vi "display.vi"() -> ()   [LabVIEW 2014]
uses:
  global variable.vi
  DataSocket/Read PLC Vars/Read U32 Var.vi
panel:
  out "选项卡控件":enum32{"选项卡 1", "选项卡 2", "选项卡 3"}(tab)
  out "Reject":i32
  out "FTT(%)":dbl format="%.1f%%"
  out "Pass":i32
  out "Actual":i32
  out "Target":dbl
  out "BTS(%)":dbl format="%.1f%%"
  out "Plan":dbl
  out "日期字符串":string
  out "时间字符串":string
  out "产品":string
  in  "生产状态":string="生产状态/Production Status"
  out "柱状图":cluster{"X轴":dbl[], "每小时产量":dbl[]}[](graph)
  out "日期字符串 2":string
  out "时间字符串 2":string
  out "产线":string
  out "日期字符串 3":string
  out "时间字符串 3":string
  out "C101":string="L541"
  out "V254":string="C53F"
  out "C101车型":string="S90L"
  out "FS11":string="CS11"
  out "FS11车型":string="领克03"
  out "V254车型":string="智道U7"
  out "FA1":string="FA1"
  # "/"
  # "/"
  # "/"
  # "/"
  # "/"
  # "/"
  # "/"
  # "/"
  # "/"
  # "/"
  # "/"
  # "/"
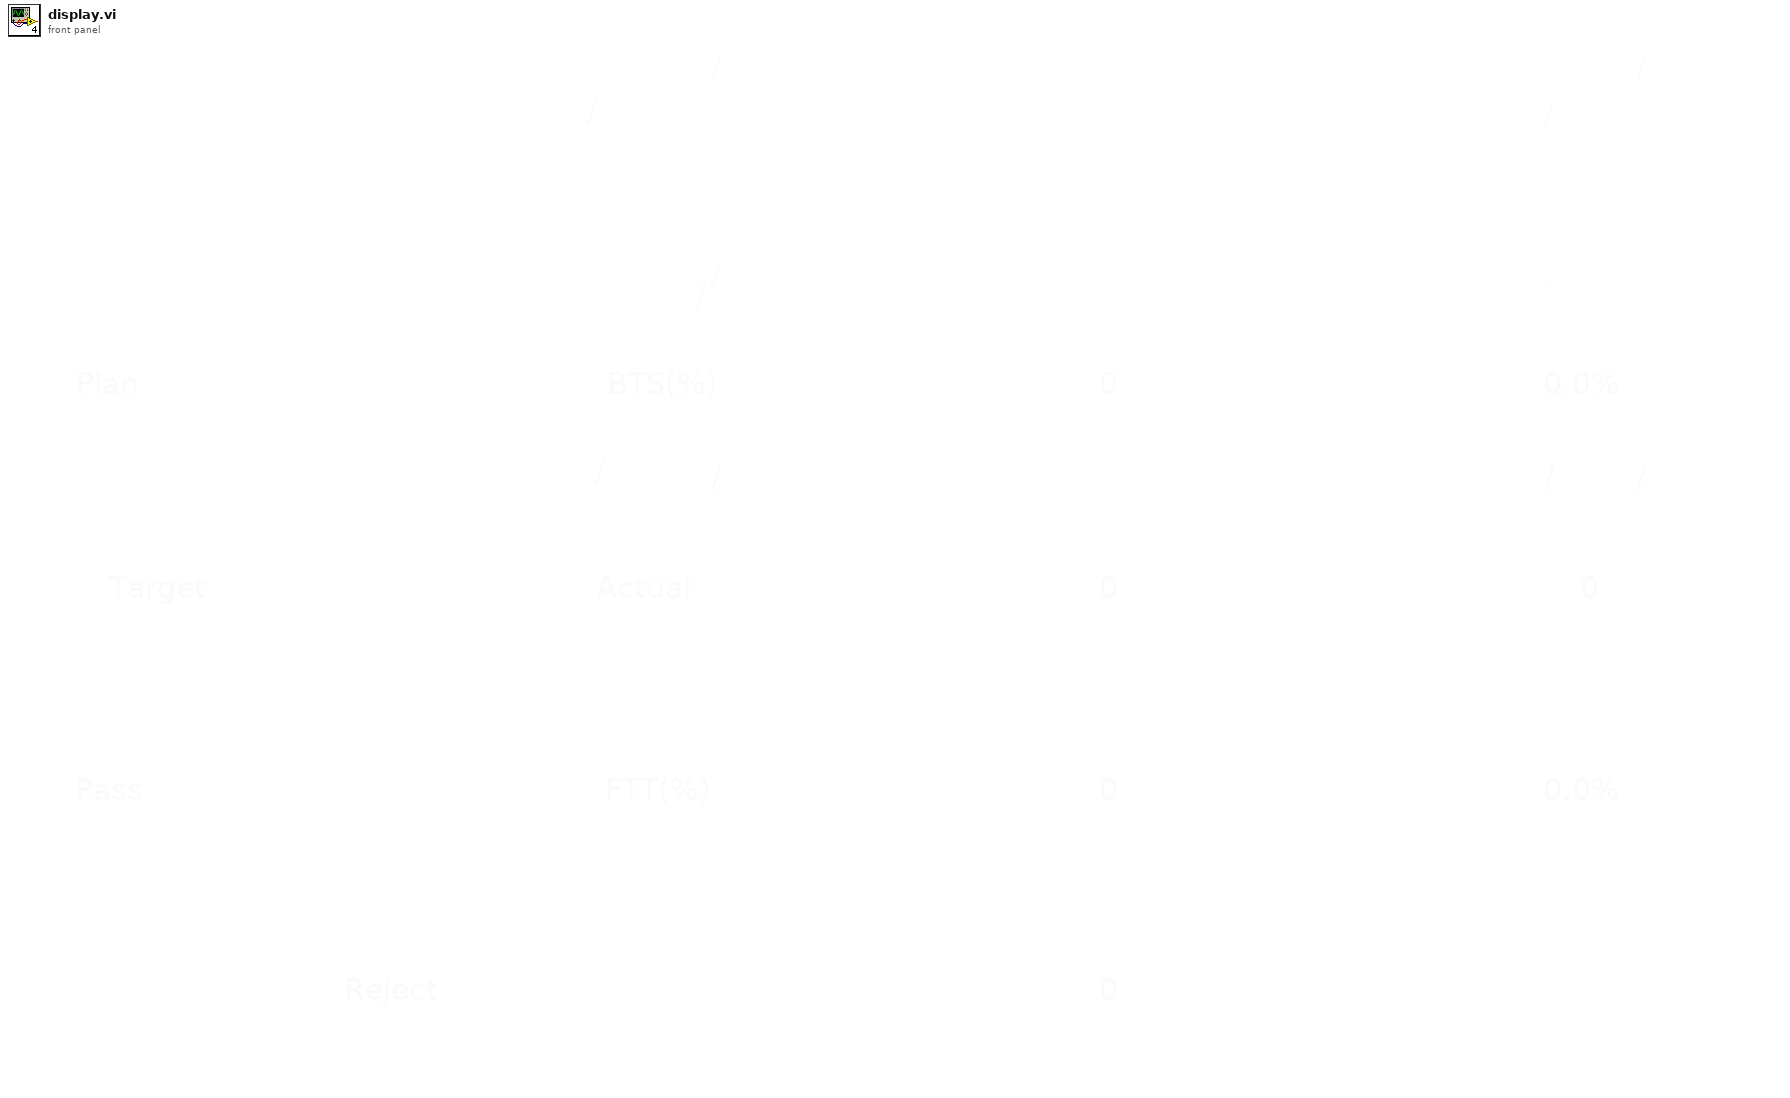
[diagram p1: front panel]
types:
  T1 = enum32{"选项卡 1", "选项卡 2", "选项卡 3", "选项卡 8", "选项卡 4", "选项卡 7", "选项卡 5", "选项卡 6"}
  T2 = typedef "DataSocket_Tags.ctl" = cluster{"Ds ID":refnum<k13>, "Tag":string}
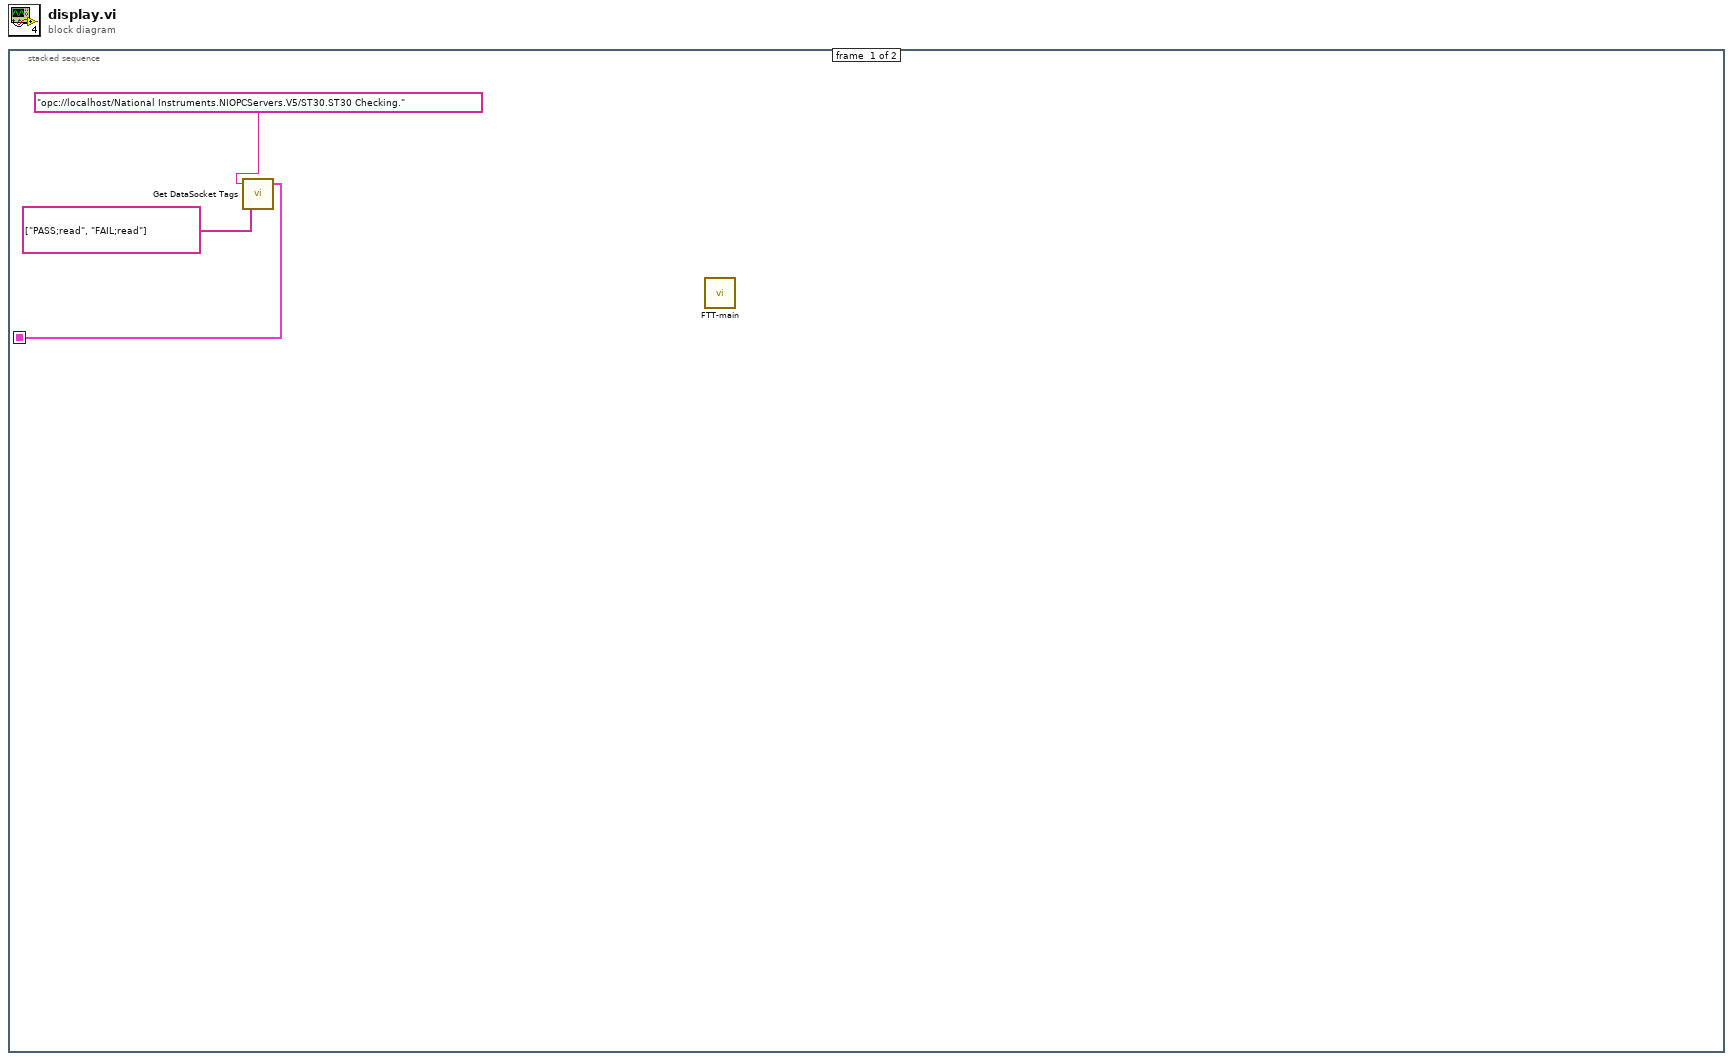
[diagram p0: block diagram]
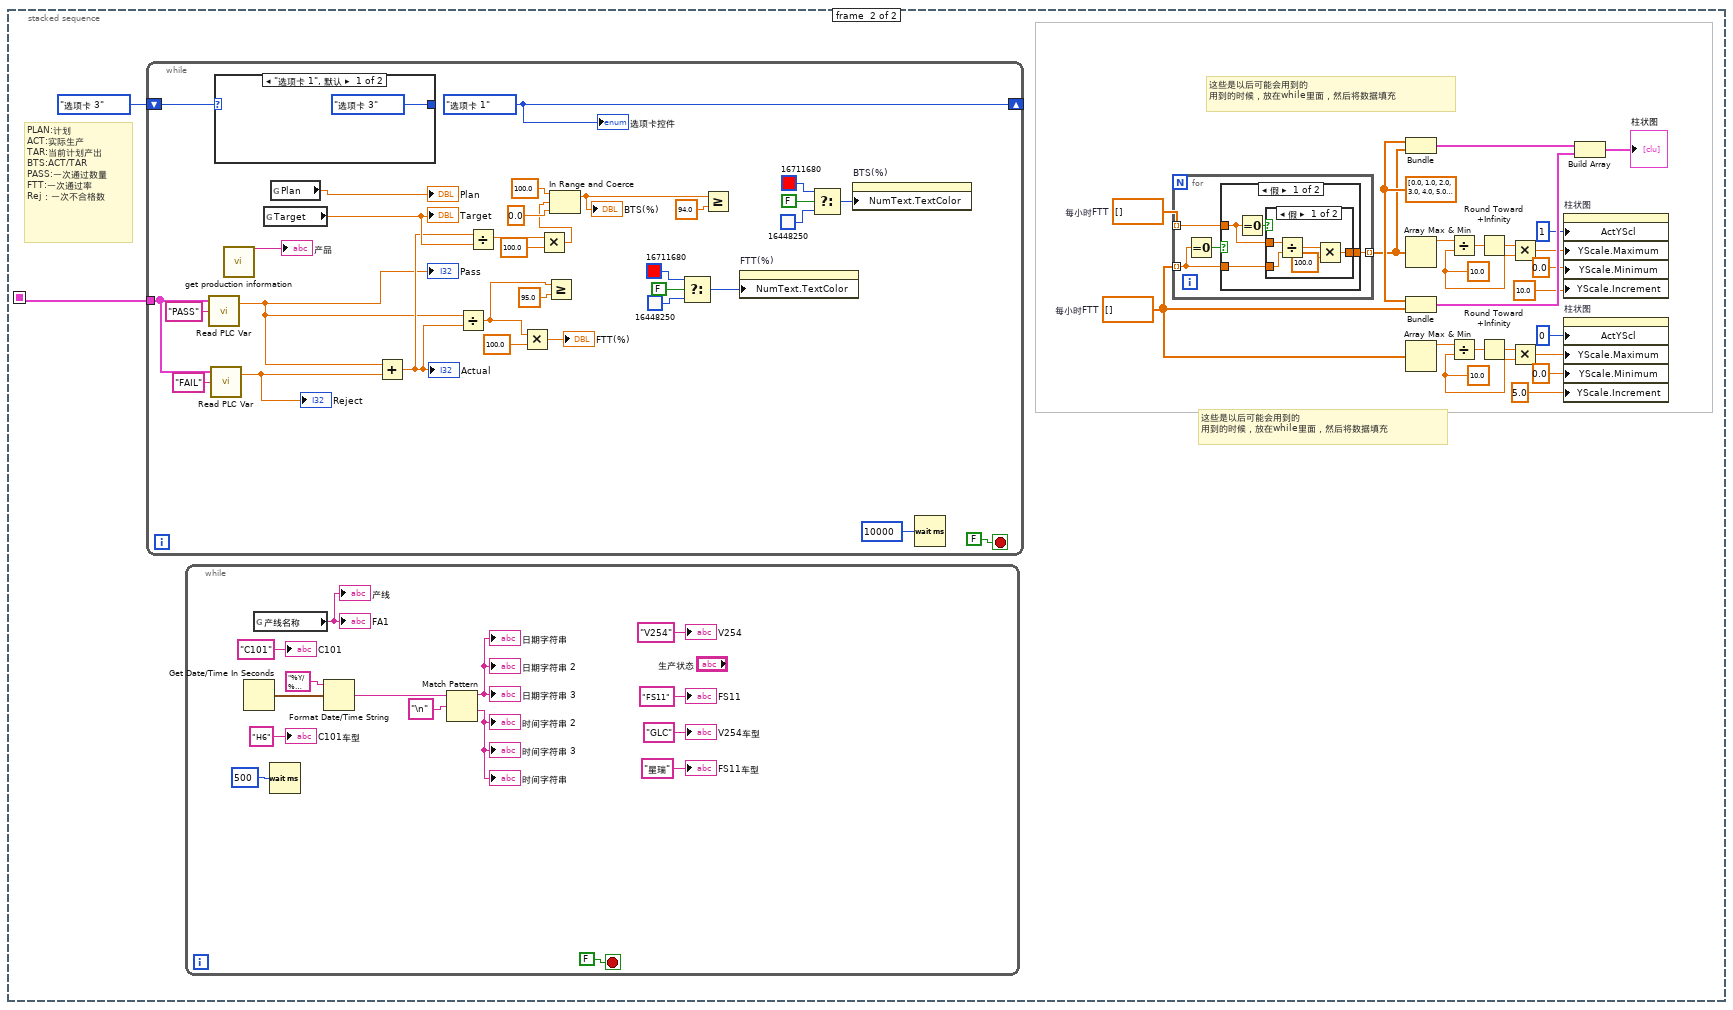
[diagram p2: hidden frame]
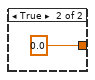
[diagram p3: hidden frame]
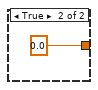
[diagram p4: hidden frame]
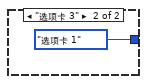
[diagram p5: hidden frame]
diagram:
  n1 = stacked-sequence {
    seq-local: [w1 _] -> [_ w4]
    frame #0 {
      n2 = call "Get DataSocket Tags.vi"("All Tags"=string[] ["PASS;read", "FAIL;read"], "URL"="opc://localhost/National Instruments.NIOPCServers.V5/ST30.ST30 Checking.") -> ("DsOut"=w1:T2[])  [unwired: 3 in]
      n3 = call "FTT-main.vi"() -> ()  [unwired: 12 in]
    }
    frame #1 {
      w27 = dbl[] []  # 每小时FTT
      w26 = dbl[] []  # 每小时FTT
      w12 = 10.0 ("y")
      w16 = 10.0 ("y")
      w22 = dbl[] [0.0, 1.0, 2.0, 3.0, 4.0, 5.0, 6.0, 7.0, 8.0, 9.0, 10.0, 11.0, 12.0, 13.0, 14.0, 15.0, 16.0, 17.0, 18.0, 19.0, 20.0, 21.0, 22.0, 23.0] ("X轴")
      # "PLAN:计划\nACT:实际生产\nTAR:当前计划产出\nBTS:ACT/TAR\nPASS:一次通过数量\nFTT:一次通过率\nRej：一次不合格数"
      # "这些是以后可能会用到的\n用到的时候，放在while里面，然后将数据填充"
      # "这些是以后可能会用到的\n用到的时候，放在while里面，然后将数据填充"
      n4 = while {
        shift-right: [w70] -> _
        shift-left: T1."选项卡 3" ("选项卡控件") -> [w87]
        tunnel: w4 -> [w62]
        stop <- FALSE stop-if-true
        w70 = T1."选项卡 1" ("选项卡控件")
        n5 = call-poly "Read PLC Var.vi"("Tag IN"="PASS", "Ds PLCTags IN"=w62) -> ("U32 Var out"=w61:dbl)  [unwired: 1 in, 1 out]
        "Pass" <- w61
        n6 = call-poly "Read PLC Var.vi"("Tag IN"="FAIL", "Ds PLCTags IN"=w62) -> ("U32 Var out"=w60:dbl)  [unwired: 1 in, 1 out]
        "Reject" <- w60
        n7 = case shown="\"选项卡 1\", 默认" w87 {
          tunnel: [T1."选项卡 3" ("选项卡控件") T1."选项卡 1" ("选项卡控件")] -> _
          frame "选项卡 1", Default {
          }
          frame "选项卡 3" {
          }
        }
        n8 = call "get production information.vi"() -> ("type"=→"产品":string)  [unwired: 9 in, 2 out]
        n9 = global read "global variable.vi" "Target"() -> (w78:dbl)
        "Target" <- w78
        n10 = global read "global variable.vi" "Plan"() -> (→"Plan":dbl)
        n11 = Add(x=w61, y=w60) -> (x+y=w77:dbl)
        "Actual" <- w77
        n12 = Divide(x=w61, y=w77) -> (x/y=w76:dbl)
        n13 = Divide(x=w77, y=w78) -> (x/y=w72:dbl)
        n14 = Multiply(x=w76, y=100.0) -> (x*y=→"FTT(%)":dbl)
        n15 = Multiply(x=w72, y=100.0) -> (x*y=w71:dbl)
        n16 = Greater Or Equal?(x=w76, y=95.0) -> ()  [unwired: 1 out]
        n17 = In Range and Coerce(upper limit=100.0 ("上限"), x=w71, lower limit=0.0 ("下限")) -> (coerced(x)=w82:dbl)  [unwired: 1 out]
        "BTS(%)" <- w82
        n18 = Select(t=u32 16711680, s=FALSE, f=u32 16448250) -> (s? t:f=w89:u32)
        n19 = Greater Or Equal?(x=w82, y=94.0) -> ()  [unwired: 1 out]
        n20 = property on="FTT(%)" class="DigNum (严格)"("NumText.TextColor"=w89) -> ()  [unwired: 2 in, 2 out]
        n21 = Select(t=u32 16711680, s=FALSE, f=u32 16448250) -> (s? t:f=w86:u32)
        n22 = property on="BTS(%)" class="DigNum (严格)"("NumText.TextColor"=w86) -> ()  [unwired: 2 in, 2 out]
        n23 = Wait (ms)(milliseconds to wait=u32 10000 ("等待时间（毫秒）")) -> ()  [unwired: 1 out]
        "选项卡控件" <- w70
      }
      n24 = while {
        stop <- FALSE stop-if-true
        n25 = Get Date/Time In Seconds() -> (seconds since 1Jan1904=w53:timestamp)
        n26 = global read "global variable.vi" "产线名称"() -> (→"产线" →"FA1":string)
        n27 = Wait (ms)(milliseconds to wait=u32 500 ("等待时间（毫秒）")) -> ()  [unwired: 1 out]
        n28 = Format Date/Time String(time format string (%c)="%Y/%m/%d\n%H:%M:%S", seconds (now)=w53) -> (date/time string=w52:string)  [unwired: 1 in]
        n29 = Match Pattern(string=w52, regular expression="\n" ("正则表达式")) -> (before substring=→"日期字符串 3" →"日期字符串" →"日期字符串 2":string, after substring=→"时间字符串 3" →"时间字符串" →"时间字符串 2":string)  [unwired: 1 in, 2 out]
        "C101" <- "C101" ("L541")
        "C101车型" <- "H6" ("S90L")
        "FS11车型" <- "星瑞" ("领克03")
        "V254车型" <- "GLC" ("智道U7")
        "FS11" <- "FS11" ("CS11")
        "V254" <- "V254" ("C53F")
      }
      n30 = for {
        tunnel: w26 -> [w31] mode=indexing
        tunnel: w27 -> [w29] mode=indexing
        tunnel: [w32] -> w11 mode=indexing
        n31 = Equal To 0?(x=w29) -> (x = 0?=w30:bool)
        n32 = case shown="假" w30 {
          tunnel: w29 -> [w36 _]
          tunnel: [w35 0.0] -> w32
          tunnel: w31 -> [w33 _]
          frame False {
            n33 = Equal To 0?(x=w33) -> (x = 0?=w34:bool)
            n34 = case shown="假" w34 {
              tunnel: w36 -> [w41 _]
              tunnel: [w38 0.0] -> w35
              tunnel: w33 -> [w37 _]
              frame False {
                n35 = Divide(x=w37, y=w41) -> (x/y=w40:dbl)
                n36 = Multiply(x=w40, y=100.0) -> (x*y=w38:dbl)
              }
              frame True {
              }
            }
          }
          frame True {
          }
        }
      }
      n37 = Bundle("X轴"=w22, w11) -> (w20:cluster{"X轴":dbl[], dbl[]})  [unwired: 1 in]
      n38 = Array Max & Min(array=w11) -> (max value=w15:dbl)  [unwired: 3 out]
      n39 = Bundle("X轴"=w22, "每小时FTT"=w27) -> (w21:cluster{"X轴":dbl[], "每小时FTT":dbl[]})  [unwired: 1 in]
      n40 = Array Max & Min(array=w27) -> (max value=w19:dbl)  [unwired: 3 out]
      n41 = Divide(x=w15, y=w12) -> (x/y=w14:dbl)
      n42 = Divide(x=w19, y=w16) -> (x/y=w18:dbl)
      n43 = Round Toward +Infinity(x=w14) -> (ceil(x): smallest int >= x=w13:dbl)
      n44 = Round Toward +Infinity(x=w18) -> (ceil(x): smallest int >= x=w17:dbl)
      n45 = Multiply(x=w13, y=w12) -> (x*y=w8:dbl)
      n46 = Multiply(x=w17, y=w16) -> (x*y=w25:dbl)
      n47 = property on="柱状图" class="XYGraph (严格)"("ActYScl"=1 ("活动Y标尺"), "YScale.Maximum"=w8, "YScale.Minimum"=0.0 ("y"), "YScale.Increment"=10.0 ("y")) -> ()  [unwired: 2 in, 2 out]
      n48 = property on="柱状图" class="XYGraph (严格)"("ActYScl"=0 ("活动Y标尺"), "YScale.Maximum"=w25, "YScale.Minimum"=0.0 ("y"), "YScale.Increment"=5.0 ("y")) -> ()  [unwired: 2 in, 2 out]
      n49 = Build Array(w20, w21) -> (→"柱状图":cluster{"X轴":dbl[], "每小时FTT":dbl[]}[])
    }
  }
